vi "detect grid for dataset.vi"(11 "Image 3":T1(plugin-control)) -> (0 "cy":dbl[](array[numeric]), 1 "cx":dbl[](array[numeric]), 2 "Circles":cluster{"x":dbl, "y":dbl, "r":dbl}[](array[cluster]), 3 "Image 4":T1(plugin-control), 4 "size(s)":i32)   [LabVIEW 2018]
panel:
  out "x":dbl[](array[numeric])
  out "y":dbl[](array[numeric])
  out "Circles (Shape Detection 1)":T2(array[cluster]) {"Position"."Y" format="%.2f"; "Position"."X" format="%.2f"}
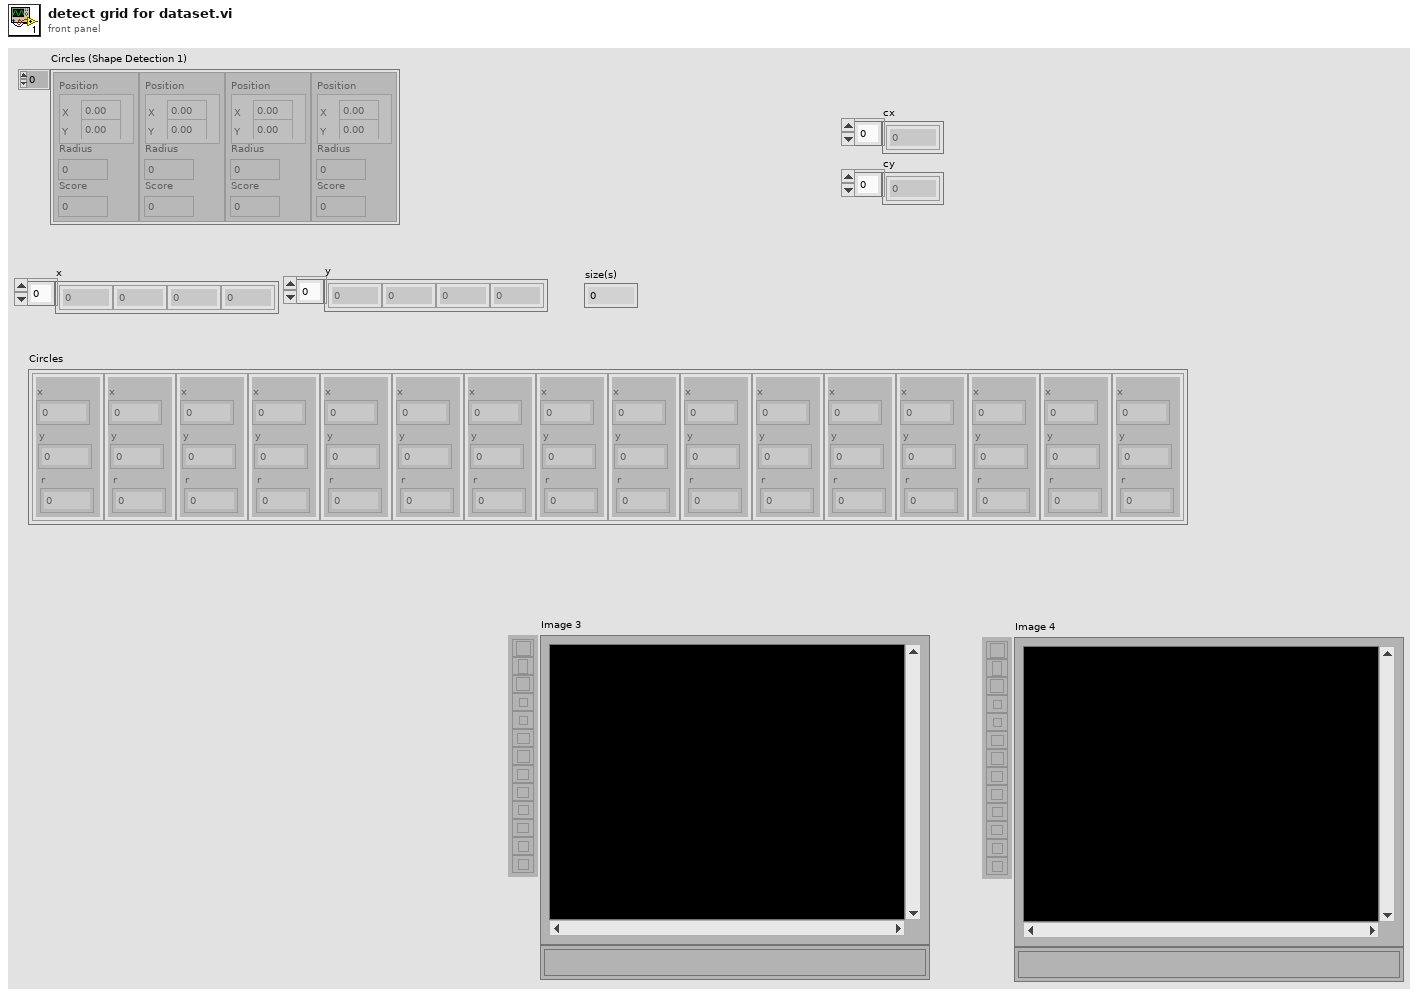
[diagram p1: front panel]
types:
  T1 = typedef "IMAQ Image.ctl" = refnum<image>
  T2 = cluster{"Position":cluster{"X":sgl, "Y":sgl}, "Radius":dbl, "Score":dbl}[]
  T3 = cluster{"Position":cluster{"X":sgl, "Y":sgl}, "Radius":dbl, "Score":dbl}
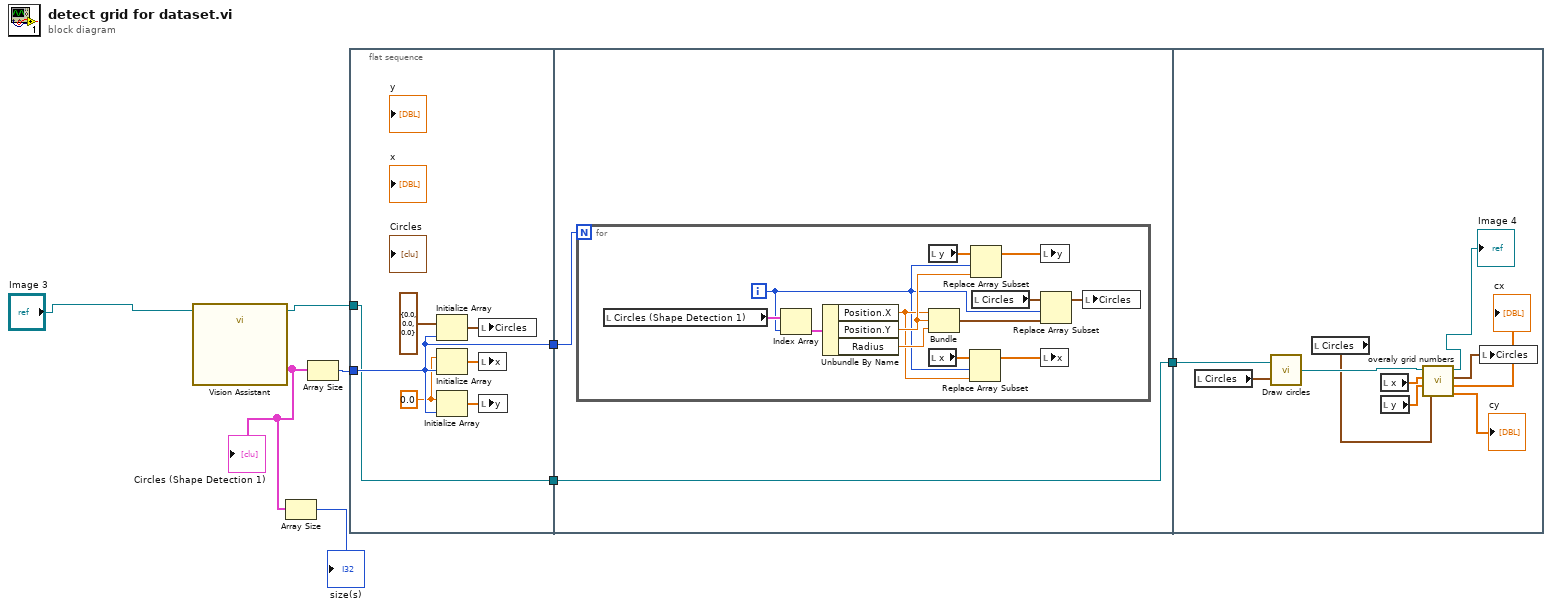
[diagram p0: block diagram]
diagram:
  n1 = call "Vision Assistant"("Image In"="Image 3") -> ("Image Out"=w4:T1, "Circles (Shape Detection 1)"=w2:T2)  [unwired: 24 in, 1 out]
  "Circles (Shape Detection 1)" <- w2
  n2 = Array Size(array=w2) -> (size(s)=→"size(s)":i32)
  n3 = Array Size(array=w2) -> (size(s)=w5:i32)
  n4 = flat-sequence {
    tunnel: [w12] -> w8
    tunnel: w5 -> [w12]
    tunnel: w4 -> [w9]
    tunnel: [w9] -> w7
    tunnel: w8 -> [w17]
    tunnel: w7 -> [w16]
    tunnel: [w16] -> w6
    tunnel: w6 -> [w35]
    frame #0 {
      w10 = 0.0 ("element")
      n5 = Initialize Array(cluster{"x":dbl, "y":dbl, "r":dbl} {"x"=0.0, "y"=0.0, "r"=0.0} ("circle"), w12) -> (w15:cluster{"x":dbl, "y":dbl, "r":dbl}[])
      n6 = Initialize Array(w10, w12) -> (w13:dbl[])
      n7 = Initialize Array(w10, w12) -> (w11:dbl[])
      n8 = local write "Circles"(w15) -> ()
      n9 = local write "x"(w13) -> ()
      n10 = local write "y"(w11) -> ()
    }
    frame #1 {
      n11 = for {
        N: w17 -> [_]
        i -> [w22]
        n12 = local read "Circles (Shape Detection 1)"() -> (w30:T2)
        n13 = Index Array(array=w30, index=w22) -> (element=w29:T3)
        n14 = Unbundle By Name(w29) -> ("Position.X"=w23:sgl, "Position.Y"=w24:sgl, "Radius"=w28:dbl)
        n15 = local read "y"() -> (w19:dbl[])
        n16 = Bundle("X"=w23, "Y"=w24, "Radius"=w28) -> (w26:cluster{"X":sgl, "Y":sgl, "Radius":dbl})  [unwired: 1 in]
        n17 = local read "x"() -> (w21:dbl[])
        n18 = Replace Array Subset(array=w21, new element=w23, index=w22) -> (w20:dbl[])
        n19 = Replace Array Subset(array=w19, new element=w24, index=w22) -> (w18:dbl[])
        n20 = local read "Circles"() -> (w27:cluster{"x":dbl, "y":dbl, "r":dbl}[])
        n21 = local write "y"(w18) -> ()
        n22 = Replace Array Subset(array=w27, new element=w26, index=w22) -> (w25:cluster{"x":dbl, "y":dbl, "r":dbl}[])
        n23 = local write "x"(w20) -> ()
        n24 = local write "Circles"(w25) -> ()
      }
    }
    frame #2 {
      n25 = local read "Circles"() -> (w40:cluster{"x":dbl, "y":dbl, "r":dbl}[])
      n26 = call "Draw circles .vi"("Circles"=w40, "Refnum in"=w35) -> ("Refnum out"=w36:T1)
      n27 = local read "Circles"() -> (w33:cluster{"x":dbl, "y":dbl, "r":dbl}[])
      n28 = local read "x"() -> (w39:dbl[])
      n29 = local read "y"() -> (w38:dbl[])
      n30 = call "overaly grid numbers.vi"("Circles"=w33, "y"=w38, "x"=w39, "Refnum in"=w36) -> ("cy"=→"cy":dbl[], "cx"=→"cx":dbl[], "Circles 2"=w37:cluster{"x":dbl, "y":dbl, "r":dbl}[], "Refnum out"=→"Image 4":T1)
      n31 = local write "Circles"(w37) -> ()
    }
  }
